vi "Shooter.vi"(0 "Shoot":bool, 1 "Feed Shooter":bool, 2 "Reverse shooter":bool, 3 "Reverse Swirly":bool, 4 "Target RPM":dbl(slide)=-0.5 scale=0.0..5000.0) -> ()   [LabVIEW 2016]
uses:
  <vilib>/Rock Robotics/WPI/ThirdParty/CanMotor/TalonSRX/WPI_CANTalonSRX_APIControlMode.ctl
  <vilib>/Rock Robotics/WPI/ThirdParty/CanMotor/TalonSRX/CTRE_CANTalonSRX_VelocityMeasurementPeriod.ctl
  <vilib>/Rock Robotics/WPI/ThirdParty/CanMotor/TalonSRX/WPI_CANTalonSRX_APIFeedbackSelect.ctl
  <vilib>/Rock Robotics/Network Tables/NT Read Number.vi
  <vilib>/Rock Robotics/Network Tables/NT Write Numeric Array.vi
panel:
  in  "NT Speed override":bool
  in  "Feeder measurement period":T1=20 items=["Period_1ms"=1, "Period_2ms"=2, "Period_5ms"=5, "Period_10ms"=10, "Period_20ms"=20, "Period_25ms"=25, "Period_50ms"=50, "Period_100ms"=100]
  in  "Feeder sample window":u32=64
  in  "Velocity Sample Window":u32=64
  in  "Velocity Measurement Period":T1=20 items=["Period_1ms"=1, "Period_2ms"=2, "Period_5ms"=5, "Period_10ms"=10, "Period_20ms"=20, "Period_25ms"=25, "Period_50ms"=50, "Period_100ms"=100]
  in  "Feeder mode":T2=enum."Speed"
  out "Feeder Speed":cluster{dbl, "Sensor Velocity":dbl}(graph)
  out "Feeder output":cluster{"Applied Throttle":dbl}(graph)
  in  "Feeder PID":T3={"P"=0.1, "I"=0.00015, "D"=0.0, "F"=0.0, "I Zone"=0.0, "Ramp Rate"=0.0}
  in  "Agitator %":dbl(slide)=1.0 scale=0.0..1.0
  in  "Shooter PID":T3={"P"=0.1, "I"=5.45e-05, "D"=0.0, "F"=0.0, "I Zone"=0.0, "Ramp Rate"=1.4}
  in  "Swirly %":dbl(slide)=0.8 scale=0.0..1.0
  out "Shooter output":cluster{"Applied Throttle":dbl}(graph)
  out "Shooter Speed":cluster{dbl, "Sensor Velocity":dbl}(graph)
  # "Figure out \nthis in RPM"
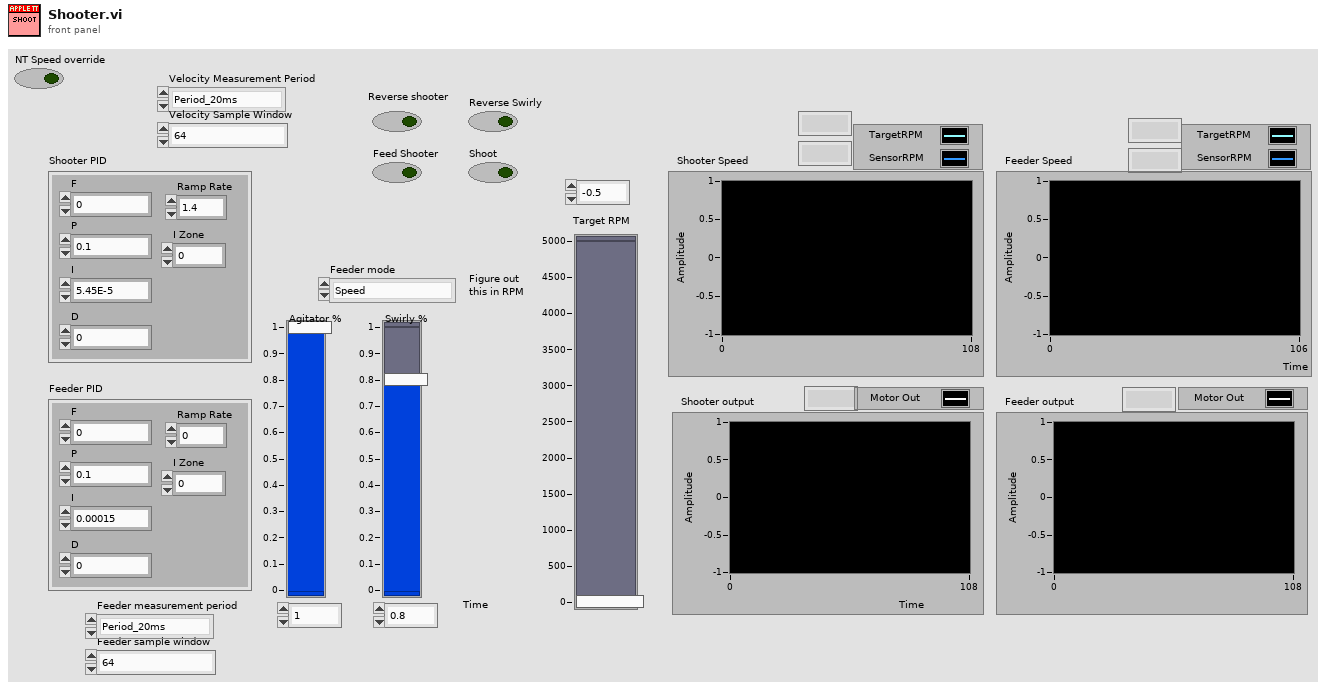
[diagram p1: front panel]
types:
  T1 = typedef "CTRE_CANTalonSRX_VelocityMeasurementPeriod.ctl" = u16
  T2 = typedef "WPI_CANTalonSRX_APIControlMode.ctl" = enum8{"Percent VBus", "Speed", "Position", "Slave", "Unchanged / Invalid", "Voltage Compensation", "Current", "Motion Profile", "Motion Magic"}
  T3 = cluster{"P":dbl, "I":dbl, "D":dbl, "F":dbl, "I Zone":dbl, "Ramp Rate":dbl}
  T4 = typedef "WPI_CANTalonSRX_APIFeedbackSelect.ctl" = enum16{"Digital Quadrature Encoder", "Analog Potentiometer", "Analog Encoder", "Count on Quad-A (Rising-Edge)", "Count on Quad-A (Falling-Edge)", "CTR Magnetic Enc (Absolute)", "CTR Magnetic Enc (Relative)", "Pulse Width"}
  T5 = typedef "WPI_MotorControlDeviceRef.ctl" = cluster{"DeviceStatus":errorcluster, "Type":T6, "PWM":cluster{"PWM Channel":T7, "DeadBand":T8}, "CAN":cluster{"Device Number":u8, "SetOutput VI Ref":variant, "GetOutput VI Ref":variant, "Enable VI Ref":variant, "Disable VI Ref":variant, "Data":variant}, "Invert":bool}
  T6 = typedef "WPI_MotorControlType.ctl" = enum16{"PWM", "CAN"}
  T7 = typedef "FPGA_DIOPWMChannel.ctl" = enum8{"PWM 0", "PWM 1", "PWM 2", "PWM 3", "PWM 4", "PWM 5", "PWM 6", "PWM 7", "PWM 8", "PWM 9", "PWM MXP 0", "PWM MXP 1", "PWM MXP 2", "PWM MXP 3", "PWM MXP 4", "PWM MXP 5", "PWM MXP 6", "PWM MXP 7", "PWM MXP 8", "PWM MXP 9", "Invalid"}
  T8 = typedef "WPI_PWMDeadband.ctl" = cluster{"Name":string, "maxPositivePwm":i32, "minPositivePwm":i32, "centerPwm":i32, "maxNegativePwm":i32, "minNegativePwm":i32, "angularRange":u16}
  T9 = typedef "WPI_CANTalonSRX_GlobalStatus.ctl" = cluster{"Applied Throttle":dbl, "Module Enabled":bool, "CAN Error":errorcluster, "Closed Loop Error":dbl, "Forward Limit Switch Closed":bool, "Reverse Limit Switch Closed":bool, "Sensor Position":dbl, "Sensor Velocity":dbl, "Current":dbl, "Sticky Fault - Over Temp":bool, "Sticky Fault - Under Voltage":bool, "Sticky Fault - Forward Limit":bool, "Sticky Fault - Reverse Limit":bool, "Sticky Fault - Forward Soft Limit":bool, "Sticky Fault - Reverse Soft Limit":bool, "Brake is Enabled":bool, "Encoder Position":dbl, "Encoder Velocity":dbl, "Encoder Index Count":dbl, "Encoder A Pin State":bool, "Encoder B Pin State":bool, "Encoder Index Pin State":bool, "Analog In":dbl, "Analog In Velocity":dbl, "Temperature (C)":dbl, "Battery Voltage":dbl, "Control 5 Is Supported":bool, "Current Profile Slot Select":dbl, "Pos Div 8":bool, "Vel Div 4":bool, "Pulse Width Position":i32, "Pulse Width Velocity":i32, "Pulse Width Rise To Rise (us)":i32, "Pulse Width Rise To Fall (us)":i32, "Mot Prof Active Is Under Run":bool, "Mot Prof Active Has Under Run":bool, "Mot Prof Active Is Last":bool, "Mot Prof Active Velocity Only":bool, "Mot Prof Active Is Valid":bool, "Mot Prof Buffer Is Full":bool, "Mot Prof Active Profile Slot Select":i32, "Mot Prof NextID":i32, "Mot Prof Count":i32, "Mot Prof Active Velocity":dbl, "Mot Prof Active Position":dbl, "Mot Prof Output Enable":i32, "UsageFrame":u32}
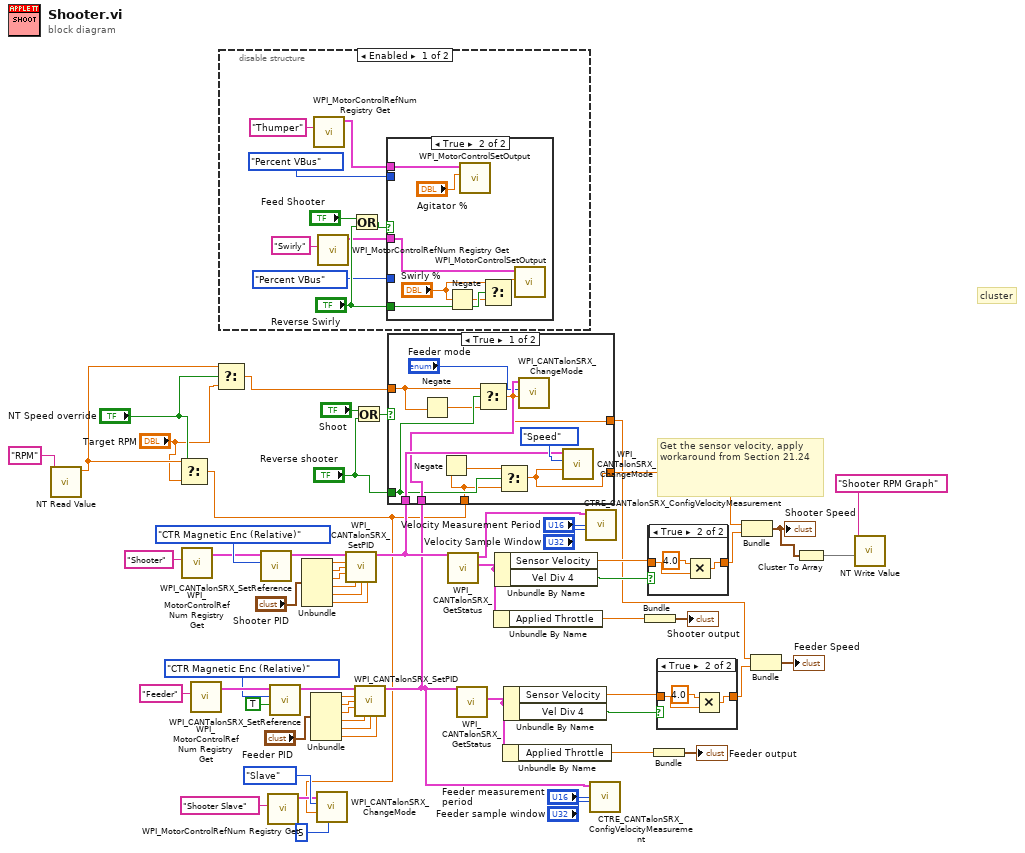
[diagram p0: block diagram]
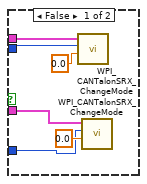
[diagram p2: hidden frame]
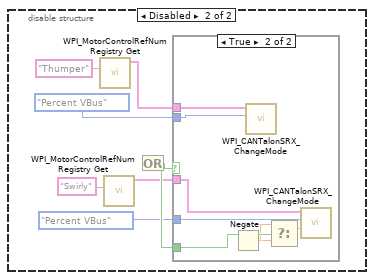
[diagram p3: hidden frame]
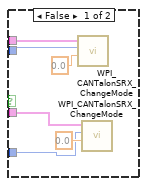
[diagram p4: hidden frame]
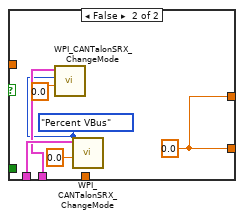
[diagram p6: hidden frame]
diagram:
  (unwired) WPI_CANTalonSRX_APIFeedbackSelect."CTR Magnetic Enc (Relative)" ("Feedback Reference Shooter")
  (unwired) "Shooter" ("refnum name")
  # "cluster"
  # "Get the sensor velocity, apply workaround from Section 21.24"
  n1 = call-poly <vilib>:"NT Read Value.vi"("Name"="RPM") -> ("Numeric"=w8:dbl)  [unwired: 9 in, 1 out]
  n2 = Select(t=w8, s="NT Speed override", f="Target RPM") -> (s? t:f=w3:dbl)
  n3 = call <vilib>:"WPI_MotorControlRefNum Registry Get.vi"("refnum name"="Shooter") -> ("MotorControlDevRef"=w57:T5)  [unwired: 9 in, 1 out]
  n4 = call <vilib>:"WPI_MotorControlRefNum Registry Get.vi"("refnum name"="Feeder") -> ("MotorControlDevRef"=w28:T5)  [unwired: 9 in, 1 out]
  n5 = Select(t=w8, s="NT Speed override", f="Target RPM") -> (s? t:f=w9:dbl)
  n6 = disable-structure shown="Enabled" {
    frame Enabled {
      n7 = call <vilib>:"WPI_MotorControlRefNum Registry Get.vi"("refnum name"="Thumper") -> ("MotorControlDevRef"=w63:T5)  [unwired: 9 in, 1 out]
      n8 = call <vilib>:"WPI_MotorControlRefNum Registry Get.vi"("refnum name"="Swirly") -> ("MotorControlDevRef"=w66:T5)  [unwired: 9 in, 1 out]
      n9 = Or(x="Feed Shooter", y="Reverse Swirly") -> (x .or. y?=w69:bool)
      n10 = case shown="True" w69 {
        tunnel: "Reverse Swirly" -> [_ w82]
        tunnel: w66 -> [w75 w79]
        tunnel: WPI_CANTalonSRX_APIControlMode."Percent VBus" ("Control Mode") -> [w74 _]
        tunnel: w63 -> [w73 w78]
        tunnel: WPI_CANTalonSRX_APIControlMode."Percent VBus" ("Control Mode") -> [w72 _]
        frame False {
          n11 = call <vilib>:"WPI_CANTalonSRX_ChangeMode.vi"("Output"=0.0, "Control Mode"=w72, "CAN Talon SRX Ref"=w73) -> ()  [unwired: 7 in, 2 out]
          n12 = call <vilib>:"WPI_CANTalonSRX_ChangeMode.vi"("Output"=0.0, "Control Mode"=w74, "CAN Talon SRX Ref"=w75) -> ()  [unwired: 7 in, 2 out]
        }
        frame True {
          n13 = Negate(x="Swirly %") -> (-x=w80:dbl)
          n14 = call <vilib>:"WPI_MotorControlSetOutput.vi"("Output"="Agitator %", "MotorControlDevRef"=w78) -> ()  [unwired: 7 in, 3 out]
          n15 = Select(t="Swirly %", s=w82, f=w80) -> (s? t:f=w83:dbl)
          n16 = call <vilib>:"WPI_MotorControlSetOutput.vi"("Output"=w83, "MotorControlDevRef"=w79) -> ()  [unwired: 7 in, 3 out]
        }
      }
    }
    frame Disabled {
      n17 = call <vilib>:"WPI_MotorControlRefNum Registry Get.vi"("refnum name"="Thumper") -> ("MotorControlDevRef"=w85:T5)  [unwired: 9 in, 1 out]
      n18 = call <vilib>:"WPI_MotorControlRefNum Registry Get.vi"("refnum name"="Swirly") -> ("MotorControlDevRef"=w88:T5)  [unwired: 9 in, 1 out]
      n19 = Or(y=w90) -> (x=w92:bool, x .or. y?=w91:bool)
      n20 = case shown="True" w91 {
        tunnel: [_ w105] -> w90
        tunnel: w88 -> [w97 w102]
        tunnel: WPI_CANTalonSRX_APIControlMode."Percent VBus" ("Control Mode") -> [w96 w101]
        tunnel: w85 -> [w95 w100]
        tunnel: WPI_CANTalonSRX_APIControlMode."Percent VBus" ("Control Mode") -> [w94 w99]
        frame False {
          n21 = call <vilib>:"WPI_CANTalonSRX_ChangeMode.vi"("Output"=0.0, "Control Mode"=w94, "CAN Talon SRX Ref"=w95) -> ()  [unwired: 7 in, 2 out]
          n22 = call <vilib>:"WPI_CANTalonSRX_ChangeMode.vi"("Output"=0.0, "Control Mode"=w96, "CAN Talon SRX Ref"=w97) -> ()  [unwired: 7 in, 2 out]
        }
        frame True {
          n23 = Negate() -> (x=w104:dbl, -x=w103:dbl)
          n24 = call <vilib>:"WPI_CANTalonSRX_ChangeMode.vi"("Control Mode"=w99, "CAN Talon SRX Ref"=w100) -> ()  [unwired: 8 in, 2 out]
          n25 = Select(t=w104, s=w105, f=w103) -> (s? t:f=w106:dbl)
          n26 = call <vilib>:"WPI_CANTalonSRX_ChangeMode.vi"("Output"=w106, "Control Mode"=w101, "CAN Talon SRX Ref"=w102) -> ()  [unwired: 7 in, 2 out]
        }
      }
    }
  }
  n27 = call <vilib>:"WPI_CANTalonSRX_SetReference.vi"("Feedback Reference"=WPI_CANTalonSRX_APIFeedbackSelect."CTR Magnetic Enc (Relative)" ("Feedback Reference Shooter"), "CAN Talon SRX Ref"=w57) -> ("CAN Talon SRX Ref"=w56:T5)  [unwired: 8 in, 1 out]
  n28 = call <vilib>:"WPI_MotorControlRefNum Registry Get.vi"("refnum name"="Shooter Slave") -> ("MotorControlDevRef"=w5:T5)  [unwired: 9 in, 1 out]
  n29 = call <vilib>:"WPI_CANTalonSRX_SetReference.vi"("Reverse Feedback Sensor"=TRUE, "Feedback Reference"=WPI_CANTalonSRX_APIFeedbackSelect."CTR Magnetic Enc (Relative)" ("Feedback Reference Shooter"), "CAN Talon SRX Ref"=w28) -> ("CAN Talon SRX Ref"=w29:T5)  [unwired: 7 in, 1 out]
  n30 = Unbundle("Shooter PID") -> ("P"=w49:dbl, "I"=w48:dbl, "D"=w47:dbl, "F"=w46:dbl, "I Zone"=w45:dbl, "Ramp Rate"=w44:dbl)
  n31 = Unbundle("Feeder PID") -> ("P"=w35:dbl, "I"=w36:dbl, "D"=w37:dbl, "F"=w38:dbl, "I Zone"=w39:dbl, "Ramp Rate"=w40:dbl)
  n32 = call <vilib>:"WPI_CANTalonSRX_ChangeMode.vi"("Master Device Number"=u8 5, "Output"=w3, "Control Mode"=WPI_CANTalonSRX_APIControlMode."Slave", "CAN Talon SRX Ref"=w5) -> ()  [unwired: 6 in, 2 out]
  n33 = call <vilib>:"WPI_CANTalonSRX_SetPID.vi"("CAN Talon SRX Ref"=w56, "P"=w49, "I"=w48, "D"=w47, "F"=w46, "I Zone"=w45, "Ramp Rate"=w44) -> ("CAN Talon SRX Ref"=w19:T5)  [unwired: 7 in, 1 out]
  n34 = Or(x="Shoot", y="Reverse shooter") -> (x .or. y?=w43:bool)
  n35 = call <vilib>:"WPI_CANTalonSRX_SetPID.vi"("CAN Talon SRX Ref"=w29, "P"=w35, "I"=w36, "D"=w37, "F"=w38, "I Zone"=w39, "Ramp Rate"=w40) -> ("CAN Talon SRX Ref"=w15:T5)  [unwired: 7 in, 1 out]
  n36 = case shown="True" w43 {
    tunnel: w19 -> [w116 w122]
    tunnel: [w114 w119] -> w52
    tunnel: "Reverse shooter" -> [w112 _]
    tunnel: w15 -> [w113 w120]
    tunnel: [w111 w119] -> w23
    tunnel: w3 -> [w109 _]
    tunnel: w9 -> [w108 _]
    frame True {
      n37 = Negate(x=w108) -> (-x=w107:dbl)
      n38 = Negate(x=w109) -> (-x=w115:dbl)
      n39 = Select(t=w108, s=w112, f=w107) -> (s? t:f=w111:dbl)
      n40 = Select(t=w115, s=w112, f=w109) -> (s? t:f=w114:dbl)
      n41 = call <vilib>:"WPI_CANTalonSRX_ChangeMode.vi"("Output"=w111, "Control Mode"="Feeder mode", "CAN Talon SRX Ref"=w113) -> ()  [unwired: 7 in, 2 out]
      n42 = call <vilib>:"WPI_CANTalonSRX_ChangeMode.vi"("Output"=w114, "Control Mode"=WPI_CANTalonSRX_APIControlMode."Speed", "CAN Talon SRX Ref"=w116) -> ()  [unwired: 7 in, 2 out]
    }
    frame False {
      w118 = WPI_CANTalonSRX_APIControlMode."Percent VBus" ("Control Mode")
      w119 = 0.0 ("x")
      n43 = call <vilib>:"WPI_CANTalonSRX_ChangeMode.vi"("Output"=0.0, "Control Mode"=w118, "CAN Talon SRX Ref"=w120) -> ()  [unwired: 7 in, 2 out]
      n44 = call <vilib>:"WPI_CANTalonSRX_ChangeMode.vi"("Output"=0.0, "Control Mode"=w118, "CAN Talon SRX Ref"=w122) -> ()  [unwired: 7 in, 2 out]
    }
  }
  n45 = call <vilib>:"WPI_CANTalonSRX_GetStatus.vi"("CAN Talon SRX Ref"=w19) -> ("Talon SRX Status"=w55:T9, "CAN Talon SRX Ref"=w18:T5)  [unwired: 8 in, 1 out]
  n46 = call <vilib>:"WPI_CANTalonSRX_GetStatus.vi"("CAN Talon SRX Ref"=w15) -> ("Talon SRX Status"=w30:T9)  [unwired: 8 in, 2 out]
  n47 = Unbundle By Name(w55) -> ("Applied Throttle"=w53:dbl)
  n48 = Unbundle By Name(w55) -> ("Sensor Velocity"=w59:dbl, "Vel Div 4"=w58:bool)
  n49 = Unbundle By Name(w30) -> ("Applied Throttle"=w32:dbl)
  n50 = Unbundle By Name(w30) -> ("Sensor Velocity"=w26:dbl, "Vel Div 4"=w27:bool)
  n51 = call <vilib>:"CTRE_CANTalonSRX_ConfigVelocityMeasurement.vi"("Velocity Sample Window"="Velocity Sample Window", "Velocity Measurement Period"="Velocity Measurement Period", "CAN Talon SRX Ref"=w18) -> ()  [unwired: 7 in, 2 out]
  n52 = call <vilib>:"CTRE_CANTalonSRX_ConfigVelocityMeasurement.vi"("Velocity Sample Window"="Feeder sample window", "Velocity Measurement Period"="Feeder measurement period", "CAN Talon SRX Ref"=w15) -> ()  [unwired: 7 in, 2 out]
  n53 = Bundle("Applied Throttle"=w53) -> (→"Shooter output":cluster{"Applied Throttle":dbl})  [unwired: 1 in]
  n54 = case shown="True" w58 {
    tunnel: [w124 w126] -> w51
    tunnel: w59 -> [w124 w125]
    frame False {
    }
    frame True {
      n55 = Multiply(x=4.0, y=w125) -> (x*y=w126:dbl)
    }
  }
  n56 = Bundle("Applied Throttle"=w32) -> (→"Feeder output":cluster{"Applied Throttle":dbl})  [unwired: 1 in]
  n57 = case shown="True" w27 {
    tunnel: [w128 w130] -> w33
    tunnel: w26 -> [w128 w129]
    frame False {
    }
    frame True {
      n58 = Multiply(x=4.0, y=w129) -> (x*y=w130:dbl)
    }
  }
  n59 = Bundle("x"=w52, "Sensor Velocity"=w51) -> (w13:cluster{"x":dbl, "Sensor Velocity":dbl})  [unwired: 1 in]
  "Shooter Speed" <- w13
  n60 = Bundle("x"=w23, "Sensor Velocity"=w33) -> (→"Feeder Speed":cluster{"x":dbl, "Sensor Velocity":dbl})  [unwired: 1 in]
  n61 = Cluster To Array(cluster=w13) -> (array=w12:dbl[])
  n62 = call-poly <vilib>:"NT Write Value.vi"("Numeric Array"=w12, "Name"="Shooter RPM Graph") -> ()  [unwired: 9 in, 1 out]
